vi "Main Tclk.vi"() -> ()   [LabVIEW 2018] (continued)
                                }
                                }
                              }
                            }
                          }
                          n5924 = local write "Status message"("Finishing FIB reheat ..." ("Status message")) -> ()
                          n5925 = local read "Stop Reheat"() -> (w964:bool)
                          n5926 = local read "Stop"() -> (w971:bool)
                          n5927 = Compound Arithmetic op=OR(w967, w971, w964) -> (w969:bool)
                        }
                      }
                      frame #5 {
                        n5928 = local read "Stop Reheat"() -> (w1024:bool)
                        n5929 = case shown="False" w1024 {
                          frame False {
                            n5930 = local read "Api"() -> (w1026:refnum<k7>)
                            n5931 = call "SmartSEM Remote API FIB HV offset removal.vi"("Max offset threshold (V)"=sgl 80.0, "Api"=w1026) -> ("FIB HV matched"=w1025:bool)  [unwired: 8 in, 1 out]
                            n5932 = local write "FIB HV target matched"(w1025) -> ()
                          }
                          frame True {
                          }
                        }
                      }
                      frame #6 {
                        n5933 = local read "Stop Reheat"() -> (w1028:bool)
                        n5934 = case shown="False" w1028 {
                          tunnel: w1029 -> [w1031 w1036]
                          frame False {
                            n5935 = local read "Reheat Output"() -> (w1034:T21)
                            n5936 = local read "FIB Reheat Log Files"() -> (w1033:path)
                            n5937 = local read "Reheat time"() -> (w1032:timestamp)
                            n5938 = local read "Capella HV Data Output"() -> (w1030:T17)
                            n5939 = local write "Status message"("FIB reheat completed" ("Status message")) -> ()
                            n5940 = call "Write FIB reheat log.vi"("Capella HV Data Output"=w1030, "Reheat Output"=w1034, "Reheat time"=w1032, "Machine Type"=w1031, "Log file path"=w1033) -> ()  [unwired: 7 in]
                          }
                          frame True {
                            n5941 = local read "Reheat Output"() -> (w1039:T21)
                            n5942 = local read "FIB Reheat Log Files"() -> (w1038:path)
                            n5943 = local read "Reheat time"() -> (w1037:timestamp)
                            n5944 = local write "Status message"("FIB reheat stopped" ("Status message")) -> ()
                            n5945 = call "Write FIB reheat log.vi"("Reheat Output"=w1039, "Reheat time"=w1037, "Machine Type"=w1036, "Log file path"=w1038) -> ()  [unwired: 8 in]
                          }
                        }
                      }
                    }
                  }
                }
              }
              frame #2 {
                w1041 = u8 0 ("FIB emission below limit counts")
                w1044 = FALSE ("Start Reheat")
                n5946 = local write "Start Reheat"(w1044) -> ()
                n5947 = local write "Stop Reheat"(w1044) -> ()
                n5948 = local write "Turn FIB Gun on"(w1044) -> ()
                n5949 = property on="Request to stop reheat" class="Bool (strict)"("DisabledEnum"=T44."Disabled and Grayed Out" ("Disabled")) -> ()  [unwired: 2 in, 2 out]
                n5950 = local write "FIB emission limit warning armed"(TRUE ("FIB emission limit warning armed")) -> ()
                n5951 = local write "FIB emission below limit counts"(w1041) -> ()
                n5952 = local write "FIB suppressor below limit counts"(w1041) -> ()
                "Reheat completed" <- TRUE ("Reheat completed")
              }
            }
          }
        }
        n5953 = local read "Stop"() -> (w768:bool)
      }
      n5954 = while {
        stop <- w5378 stop-if-true
        n5955 = stacked-sequence {
          tunnel: [_ w5424] -> w5378
          frame #0 {
            n5956 = local read "Spot"() -> (w5381:bool)
            n5957 = shared-variable "My Computer\\Zeiss Library.lvlib\\Spot"(w5381) -> ()  [unwired: 1 in, 1 out]
            n5958 = local read "Machine Type"() -> (w5380:u8)
            n5959 = case shown="True" w5381 {
              tunnel: w5380 -> [_ w5383]
              frame False {
                n5960 = shared-variable ".\\Zeiss Library.lvlib\\FIB spot mode"(FALSE ("FIB spot mode")) -> ()  [unwired: 1 in, 1 out]
              }
              frame True {
                n5961 = stacked-sequence {
                  tunnel: w5383 -> [_ _ _ _ w5405 _ _]
                  frame #0 {
                    w5385 = 5.0 ("Cursor.Cursor Position:Cursor X")
                    w5384 = FALSE ("Unfreeze")
                    w5386 = TRUE ("Realtime Imaging stop")
                    n5962 = shared-variable "My Computer\\Zeiss Library.lvlib\\Realtime Imaging stop"(w5386) -> ()  [unwired: 1 in, 1 out]
                    n5963 = shared-variable ".\\Zeiss Library.lvlib\\FIB spot mode"(w5386) -> ()  [unwired: 1 in, 1 out]
                    n5964 = property on="FIB Imaging" class="Bool (strict)"("DisabledEnum"=T44."Disabled and Grayed Out" ("Disabled")) -> ()  [unwired: 2 in, 2 out]
                    n5965 = property on="FIB Image" class="IntGraph (strict)"() -> ("Width"=w5388:u32, "Height"=w5389:u32)  [unwired: 2 in, 2 out]
                    n5966 = expression code="x/2"(w5388) -> ()  [unwired: 1 out]
                    n5967 = expression code="x/2"(w5389) -> ()  [unwired: 1 out]
                    n5968 = local write "FIB Imaging"(w5384) -> ()
                    n5969 = local write "Unfreeze"(w5384) -> ()
                    n5970 = property on="FIB Image" class="IntGraph (strict)"("Cursor.Cursor X"=w5385, "Cursor.Cursor Y"=w5385) -> ()  [unwired: 2 in, 2 out]
                  }
                  frame #1 {
                    w5390 = -0.99 ("Spot X")
                    n5971 = Wait (ms)(milliseconds to wait=u32 500) -> ()  [unwired: 1 out]
                    n5972 = shared-variable ".\\Zeiss Library.lvlib\\Spot X"(w5390) -> ()  [unwired: 1 in, 1 out]
                    n5973 = shared-variable "My Computer\\Zeiss Library.lvlib\\Spot Z"(w5390) -> ()  [unwired: 1 in, 1 out]
                  }
                  frame #2 {
                    n5974 = local read "FIB HW Config"() -> (w5393:T23)
                    n5975 = local read "FIB Options"() -> (w5397:T33)
                    n5976 = local read "FIB Scan Parameters"() -> (w5392:T32)
                    n5977 = Unbundle By Name(w5397) -> ("Flip x"=w5396:bool, "Flip z"=w5395:bool)
                    n5978 = Bundle("Flip x"=w5396, "Flip z"=w5395) -> (w5394:cluster{"Flip x":bool, "Flip z":bool})  [unwired: 1 in]
                    n5979 = call "FIB spot PXIe-6124.vi"("FIB Scan Parameters"=w5392, "Options"=w5394, "HW Config"=w5393) -> ("error out"=w5399:errorcluster)  [unwired: 8 in]
                    n5980 = Unbundle By Name(w5399) -> ("status"=w5398:bool)
                    n5981 = case shown="True" w5398 {
                      frame False {
                      }
                      frame True {
                        n5982 = local write "Spot"(FALSE ("Spot")) -> ()
                      }
                    }
                  }
                  frame #3 {
                    n5983 = disable-structure shown="Disabled" {
                      frame Disabled {
                        w5404 = TRUE ("Unfreeze")
                        n5984 = local write "FIB Imaging"(w5404) -> ()
                        n5985 = local write "Unfreeze"(w5404) -> ()
                      }
                      frame Enabled {
                      }
                    }
                    n5986 = shared-variable ".\\Zeiss Library.lvlib\\FIB spot mode"(FALSE ("Realtime Imaging stop")) -> ()  [unwired: 1 in, 1 out]
                    n5987 = property on="FIB Imaging" class="Bool (strict)"("DisabledEnum"=T44."Enabled" ("Disabled")) -> ()  [unwired: 2 in, 2 out]
                    n5988 = property on="Spot" class="Bool (strict)"("DisabledEnum"=T44."Disabled and Grayed Out" ("Disabled")) -> ()  [unwired: 2 in, 2 out]
                  }
                  frame #4 {
                    n5989 = case shown="2" w5405 {
                      frame 0, Default {
                      }
                      frame 1 {
                        w5407 = TRUE ("Initialization")
                        n5990 = local read "COM port"() -> (w5406:refnum<visa-resource-name>)
                        n5991 = call "FIB mode.vi"("Initialization"=w5407, "FIB mode"=T10."SEM", "COM port in"=w5406) -> ("COM port out"=w5412:refnum<visa-resource-name>)  [unwired: 7 in, 1 out]
                        n5992 = call "Remcon32 command.vi"("SEM command"="edx 0", "COM port in"=w5412) -> ("COM port out"=w5411:refnum<visa-resource-name>)  [unwired: 6 in, 3 out]
                        n5993 = call "Remcon32 command.vi"("Close session"=w5407, "SEM command"="frez", "COM port in"=w5411) -> ()  [unwired: 5 in, 4 out]
                      }
                      frame 2 {
                        n5994 = local read "Api"() -> (w5413:refnum<k7>)
                        n5995 = call "SmartSEM Remote API set float.vi"("vValue"=sgl 2.0, "lpszParam"="DP_FIB_BLANKER_MODE" ("lpszCommand"), "Api"=w5413) -> ("error out"=w5421:errorcluster, "Api out"=w5420:refnum<k7>)  [unwired: 7 in]
                        n5996 = call "SmartSEM Remote API FIB mode.vi"("error in"=w5421, "FIB mode"=T50."SEM", "Api"=w5420) -> ("error out"=w5417:errorcluster, "Api out"=w5416:refnum<k7>)  [unwired: 7 in]
                        n5997 = invoke class="_EMApi" method="Execute"(reference=w5416, error in=w5417, "lpszCommand"="CMD_FREEZE_ALL") -> ()  [unwired: 1 in, 4 out]
                      }
                    }
                  }
                  frame #5 {
                    n5998 = Wait (ms)(milliseconds to wait=u32 4000) -> ()  [unwired: 1 out]
                  }
                  frame #6 {
                    n5999 = property on="Spot" class="Bool (strict)"("DisabledEnum"=T44."Enabled" ("Disabled")) -> ()  [unwired: 2 in, 2 out]
                  }
                }
              }
            }
          }
          frame #1 {
            n6000 = local read "Stop"() -> (w5424:bool)
          }
        }
        n6001 = Wait Until Next ms Multiple(millisecond multiple=u32 100) -> ()  [unwired: 1 out]
      }
      n6002 = while {
        stop <- w2345 stop-if-true
        n6003 = case shown="True" "Scan xn" {
          tunnel: [w2347 w2348] -> w2345
          frame False {
            n6004 = local read "Stop"() -> (w2347:bool)
          }
          frame True {
            n6005 = while {
              tunnel: [w2351] -> w2348
              stop <- w2353 stop-if-true
              n6006 = stacked-sequence {
                seq-local: [w2355 _ _ _] -> [_ w2371 _ _]
                seq-local: [_ w2370 _ _] -> [_ _ w2377 _]
                seq-local: [_ w2369 _ _] -> [_ _ w2378 _]
                frame #0 {
                  n6007 = local read "Tiled scan inputs"() -> (w2356:T6)
                  n6008 = local read "SEM HW Config"() -> (w2357:T9)
                  n6009 = local read "Detector Information"() -> (w2358:T8)
                  n6010 = local read "SEM Scan Parameters"() -> (w2359:T26)
                  n6011 = local read "SEM Options"() -> (w2360:T27)
                  n6012 = local read "Focus Index Options"() -> (w2354:T28)
                  n6013 = local read "File Information"() -> (w2361:T31)
                  n6014 = local read "Milling para"() -> (w2362:T35)
                  n6015 = Bundle By Name(cluster=w2356, "HW Config"=w2357, "Det Info"=w2358, "SEM Scan Parameters"=w2359, "SEM Options"=w2360, "Focus Index Options"=w2354, "File Information"=w2361, "Milling para"=w2362) -> (w2355:T6)
                }
                frame #1 {
                  n6016 = call "2D scan tiled.vi"("Tiled scan inputs"=w2371) -> ("Image Focus Index Tiled"=w2369:T52, "Image Focus Index Array Tiled"=w2370:T53, "Single scan outputs"=w2374:T54, "8-bit over scale"=w2363:bool[])  [unwired: 5 in, 2 out]
                  n6017 = Unbundle By Name(w2374) -> ("SEM Parameters"=w2373:T13, "Image Focus Index"=w2372:T14)
                  n6018 = Index Array(array=w2363, index #1=0 ("index"), index #2=1 ("index")) -> (element #1=w2366:bool, element #2=w2367:bool)
                  n6019 = local write "SEM Parameters"(w2373) -> ()
                  n6020 = local write "Image Focus Index"(w2372) -> ()
                  n6021 = local write "Det A over scale"(w2366) -> ()
                  n6022 = local write "Det B over scale"(w2367) -> ()
                  n6023 = local write "Status message"("SEM scanning" ("Status message")) -> ()
                }
                frame #2 {
                  n6024 = local read "FI Detector"() -> (w2379:u16)
                  n6025 = case shown="0, Default" w2379 {
                    tunnel: w2378 -> [w2383 w2387 w2391 w2395]
                    tunnel: [w2382 w2384 w2390 w2394] -> w2376
                    tunnel: w2377 -> [w2380 w2386 w2389 w2393]
                    tunnel: [w2381 w2385 w2388 w2392] -> w2375
                    frame 0, Default {
                      n6026 = Unbundle By Name(w2383) -> ("A Img Focus Index"=w2382:sgl[][])
                      n6027 = Unbundle By Name(w2380) -> ("A Img Focus Index array"=w2381:sgl[][][][])
                    }
                    frame 1 {
                      n6028 = Unbundle By Name(w2387) -> ("B Img Focus Index"=w2384:sgl[][])
                      n6029 = Unbundle By Name(w2386) -> ("B Img Focus Index array"=w2385:sgl[][][][])
                    }
                    frame 2 {
                      n6030 = Unbundle By Name(w2391) -> ("C Img Focus Index"=w2390:sgl[][])
                      n6031 = Unbundle By Name(w2389) -> ("C Img Focus Index array"=w2388:sgl[][][][])
                    }
                    frame 3 {
                      n6032 = Unbundle By Name(w2395) -> ("D Img Focus Index"=w2394:sgl[][])
                      n6033 = Unbundle By Name(w2393) -> ("D Img Focus Index array"=w2392:sgl[][][][])
                    }
                  }
                  n6034 = local write "Focus Index array tiled"(w2375) -> ()
                  n6035 = local write "Focus Index tiled"(w2376) -> ()
                }
                frame #3 {
                  n6036 = local read "Scan xn"() -> (w2396:bool)
                  n6037 = case shown="False" w2396 {
                    tunnel: ["SEM scanning pause" ("Status message") "SEM scanning finished" ("Status message")] -> w2397
                    frame True {
                    }
                    frame False {
                    }
                  }
                  n6038 = local write "Status message"(w2397) -> ()
                  n6039 = Wait (ms)(milliseconds to wait=u32 1000) -> ()  [unwired: 1 out]
                }
              }
              n6040 = Wait Until Next ms Multiple(millisecond multiple=u32 100) -> ()  [unwired: 1 out]
              n6041 = local read "Scan xn"() -> (w2352:bool)
              n6042 = Not(x=w2352) -> (.not. x?=w2350:bool)
              n6043 = local read "Stop"() -> (w2351:bool)
              n6044 = Or(x=w2350, y=w2351) -> (x .or. y?=w2353:bool)
            }
          }
        }
        n6045 = Wait Until Next ms Multiple(millisecond multiple=u32 100) -> ()  [unwired: 1 out]
      }
      n6046 = while {
        stop <- w2927 stop-if-true
        w2934 = -1.0 ("lower limit")
        w2935 = 1.0 ("upper limit")
        n6047 = property on="FIB Image" class="IntGraph (strict)"() -> ("Cursor.Cursor X"=w2929:dbl, "Width"=w2928:u32, "Cursor.Cursor Y"=w2931:dbl, "Height"=w2930:u32)  [unwired: 2 in, 2 out]
        n6048 = local read "Stop"() -> (w2927:bool)
        n6049 = Wait Until Next ms Multiple(millisecond multiple=u32 10) -> ()  [unwired: 1 out]
        n6050 = Not(x=w2927) -> (.not. x?=w2925:bool)
        n6051 = expression code="x/2"(w2928) -> (w2933:u32)
        n6052 = expression code="x/2"(w2930) -> (w2932:u32)
        n6053 = Compound Arithmetic op=AND("Spot", w2925) -> (w2945:bool)
        n6054 = shared-variable "My Computer\\Zeiss Library.lvlib\\Milling Manual Pause"("Mill Manual Pause") -> (error out=w2924:errorcluster)  [unwired: 1 in]
        n6055 = shared-variable "My Computer\\Zeiss Library.lvlib\\Milling Stop"("Mill Stop", error in=w2924) -> (error out=w2923:errorcluster)
        n6056 = shared-variable ".\\Zeiss Library.lvlib\\FIB beam blank"("Beam blanked", error in=w2923) -> (error out=w2922:errorcluster)
        n6057 = property on="FIB Image" class="IntGraph (strict)"("Cursor.Visible"="Spot") -> ()  [unwired: 2 in, 2 out]
        n6058 = Subtract(x=w2929, y=w2933) -> (x-y=w2941:dbl)
        n6059 = Subtract(x=w2931, y=w2932) -> (x-y=w2940:dbl)
        n6060 = Divide(x=w2941, y=w2933) -> (x/y=w2939:dbl)
        n6061 = Divide(x=w2940, y=w2932) -> (x/y=w2936:dbl)
        n6062 = In Range and Coerce(upper limit=w2935, x=w2939, lower limit=w2934) -> (coerced(x)=w2938:dbl)  [unwired: 1 out]
        n6063 = In Range and Coerce(upper limit=w2935, x=w2936, lower limit=w2934) -> (coerced(x)=w2937:dbl)  [unwired: 1 out]
        n6064 = shared-variable ".\\Zeiss Library.lvlib\\Spot X"(w2938, error in=w2922) -> (error out=w2921:errorcluster)
        n6065 = shared-variable "My Computer\\Zeiss Library.lvlib\\Spot Z"(w2937, error in=w2921) -> (error out=w2920:errorcluster)
        n6066 = shared-variable ".\\Zeiss Library.lvlib\\FIB spot mode"(w2945, error in=w2920) -> ()  [unwired: 1 out]
      }
      n6067 = while {
        stop <- w5362 stop-if-true
        n6068 = case shown="True" "Mill" {
          frame False {
            n6069 = property on="FIB Imaging" class="Bool (strict)"("DisabledEnum"=T44."Enabled" ("Disabled")) -> ()  [unwired: 2 in, 2 out]
          }
          frame True {
            n6070 = stacked-sequence {
              frame #0 {
                w5365 = FALSE ("Freeze")
                n6071 = local write "Unfreeze"(w5365) -> ()
                n6072 = local write "Mill Manual Pause"(w5365) -> ()
                n6073 = local write "Mill Stop"(w5365) -> ()
              }
              frame #1 {
                n6074 = Wait (ms)(milliseconds to wait=u32 500) -> ()  [unwired: 1 out]
              }
              frame #2 {
                n6075 = local read "FIB HW Config"() -> (w5371:T23)
                n6076 = local read "FIB Scan Parameters"() -> (w5370:T32)
                n6077 = local read "FIB Options"() -> (w5375:T33)
                n6078 = local read "Machine Type"() -> (w5368:u8)
                n6079 = Unbundle By Name(w5375) -> ("Flip x"=w5374:bool, "Flip z"=w5373:bool)
                n6080 = local read "COM port"() -> (w5369:refnum<visa-resource-name>)
                n6081 = Bundle("Flip x"=w5374, "Flip z"=w5373) -> (w5372:cluster{"Flip x":bool, "Flip z":bool})  [unwired: 1 in]
                n6082 = call "FIB trapezoidal mill PXIe-6124.vi"("Machine Type"=w5368, "COM port"=w5369, "Milling para"="Milling para", "Options"=w5372, "FIB Scan Parameters"=w5370, "HW Config"=w5371) -> ()  [unwired: 2 in, 4 out]
              }
              frame #3 {
                n6083 = shared-variable "My Computer\\Zeiss Library.lvlib\\Milling Line Paused"(TRUE ("Rect Milling Line Paused")) -> ()  [unwired: 1 in, 1 out]
                n6084 = local write "Mill"(FALSE ("Mill")) -> ()
              }
            }
          }
        }
        n6085 = Wait Until Next ms Multiple(millisecond multiple=u32 100) -> ()  [unwired: 1 out]
        n6086 = local read "Stop"() -> (w5362:bool)
      }
      n6087 = while {
        stop <- w1769 stop-if-true
        n6088 = Wait Until Next ms Multiple(millisecond multiple=u32 100) -> ()  [unwired: 1 out]
        n6089 = case shown="True" "Enable logging" {
          frame False {
          }
          frame True {
            n6090 = stacked-sequence {
              frame #0 {
                n6091 = Get Date/Time In Seconds() -> (seconds since 1Jan1904=w1775:timestamp)
                n6092 = Reciprocal(x="Sample rate (Hz)") -> (1/x=w1772:dbl)
                n6093 = To Double Precision Float(number=w1775) -> (double precision float=w1774:dbl)
                n6094 = property on="Measurements" class="WFChart (strict)"("History Data"=dbl[][] [], "XScale.Offset"=w1774, "XScale.Multiplier"=w1772) -> ()  [unwired: 2 in, 2 out]
              }
              frame #1 {
                w1790 = 10123 items=["Finite Samples"=10178, "Continuous Samples"=10123, "Hardware Timed Single Point"=12522] ("sample mode")
                n6095 = local read "Sample rate (Hz)"() -> (w1780:dbl)
                n6096 = local read "Active logging channels"() -> (w1779:string)
                n6097 = call-poly <vilib>:"DAQmx Create Virtual Channel.vi"("physical channels"=w1779) -> ("task out"=w1789:refnum<k21>, "error out"=w1788:errorcluster)  [unwired: 13 in]
                n6098 = call-poly <vilib>:"DAQmx Timing.vi"("task/channels in"=w1789, "sample mode"=w1790, "rate"=w1780, "error in"=w1788) -> ("task out"=w1777:refnum<k21>, "error out"=w1786:errorcluster)  [unwired: 10 in]
                n6099 = local read "Machine Type"() -> (w1776:u8)
                n6100 = call <vilib>:"DAQmx Configure Input Buffer.vi"("task/channels in"=w1777, "buffer size (in samples per channel)"=u32 1000000, "error in"=w1786) -> ("task out"=w1787:refnum<k21>, "error out"=w1785:errorcluster)  [unwired: 11 in]
                n6101 = call <vilib>:"DAQmx Start Task.vi"("task/channels in"=w1787, "error in"=w1785) -> ("task out"=w1782:refnum<k21>, "error out"=w1781:errorcluster)  [unwired: 12 in]
                n6102 = while {
                  tunnel: w1781 -> [w1820]
                  tunnel: w1782 -> [w1819]
                  tunnel: [w1818] -> w1783
                  tunnel: [w1817] -> w1784
                  tunnel: w1776 -> [w1795]
                  stop <- w1813 stop-if-true
                  n6103 = local read "Faraday Cup before mill"() -> (w1802:sgl)
                  n6104 = call-poly <vilib>:"DAQmx Read.vi"("task/channels in"=w1819, "number of samples per channel"="Samples size", "error in"=w1820) -> ("task out"=w1818:refnum<k21>, "data"=w1811:dbl[][], "error out"=w1817:errorcluster)  [unwired: 10 in]
                  n6105 = To Single Precision Float(number=w1811) -> (single precision float=w1810:sgl[][])
                  n6106 = expression code="x*10"(w1810) -> (w1793:sgl[][])
                  n6107 = case shown="2" w1795 {
                    tunnel: w1793 -> [w1821 w1824]
                    tunnel: "Samples size" -> [_ w1823]
                    tunnel: [w1821 w1822] -> w1792
                    frame 0, Default {
                    }
                    frame 2 {
                      n6108 = local read "Api"() -> (w1825:refnum<k7>)
                      n6109 = call "SmartSEM Remote API FIB Faraday cup.vi"("Api"=w1825) -> ("FIB Faraday Cup (nA)"=w1826:sgl)  [unwired: 8 in, 2 out]
                      n6110 = Initialize Array(w1826, w1823) -> (w1827:sgl[])
                      n6111 = Replace Array Subset(array=w1824, new element=w1827) -> (w1822:sgl[][])  [unwired: 2 in]
                    }
                  }
                  "Measurements" <- w1792
                  n6112 = call "2D Array Decimate.vi"("x decimating factor"="Samples size", "Input 2D Array"=w1792) -> ("output array"=w1809:dbl[][])  [unwired: 7 in, 2 out]
                  n6113 = To Single Precision Float(number=w1809) -> (single precision float=w1808:sgl[][])
                  n6114 = Index Array(array=w1808, index (col)=0 ("disabled index (col)")) -> (element=w1804:sgl[])  [unwired: 1 in]
                  n6115 = Index Array(array=w1804, index #1=3 ("index"), index #2=2 ("index"), index #3=1 ("index"), index #4=0 ("index")) -> (element #1=→"BD2 RT":sgl, element #2=w1801:sgl, element #3=→"Specimen RT":sgl, element #4=→"Faraday Cup RT":sgl)
                  "BD1 RT" <- w1801
                  n6116 = local read "Enable logging"() -> (w1816:bool)
                  n6117 = Subtract(x=w1802, y=w1801) -> (x-y=w1805:sgl)
                  n6118 = local read "Stop"() -> (w1814:bool)
                  n6119 = Build Array (concatenate)(w1804, w1805) -> (w1803:sgl[])
                  n6120 = shared-variable ".\\Zeiss Library.lvlib\\Logs"(w1803) -> ()  [unwired: 1 in, 1 out]
                  n6121 = Not(x=w1816) -> (.not. x?=w1815:bool)
                  n6122 = Or(x=w1815, y=w1814) -> (x .or. y?=w1813:bool)
                }
                n6123 = call <vilib>:"DAQmx Clear Task.vi"("task in"=w1783, "error in"=w1784) -> ("error out"=w1778:errorcluster)  [unwired: 13 in]
                n6124 = call <vilib>:"General Error Handler.vi"("error in (no error)"=w1778) -> ()  [unwired: 10 in, 5 out]
              }
            }
          }
        }
        n6125 = local read "Stop"() -> (w1769:bool)
      }
      n6126 = while {
        shift-right: [w1829] -> _
        shift-left: _ -> [w1828]
        stop <- w1831 stop-if-true
        n6127 = stacked-sequence {
          tunnel: [_ _ _ _ _ _ _ _ _ _ _ _ _ _ _ _ w2138 _ _ _ _ _ _ _ _ _] -> w1829
          tunnel: w1828 -> [_ _ _ _ _ _ _ _ _ _ _ _ _ _ _ _ w2139 w2156 w2174 _ _ _ _ _ _ _]
          frame #0 {
            n6128 = local read "FIB slice #"() -> (w1836:u32)
            n6129 = Not Equal To 0?(x="Images per Auto Optimization") -> (x != 0?=w1833:bool)
            n6130 = Not Equal To 0?(x=w1836) -> (x != 0?=w1837:bool)
            n6131 = Compound Arithmetic op=AND("Auto Optimzation", w1833, w1837) -> (w1832:bool)
            n6132 = case shown="True" w1832 {
              frame False {
              }
              frame True {
                n6133 = local read "WD array tiled"() -> (w1843:sgl[][][])
                n6134 = local read "StigX array tiled"() -> (w1841:sgl[][][])
                n6135 = local read "StigY array tiled"() -> (w1840:sgl[][][])
                n6136 = local read "AF Steps"() -> (w1859:u8)
                n6137 = local read "FIB slice #"() -> (w1853:u32)
                n6138 = local read "Images per Auto Optimization"() -> (w1857:u16)
                n6139 = Empty Array?(array=w1843) -> (empty?=w1842:bool)
                n6140 = Empty Array?(array=w1841) -> (empty?=w1839:bool)
                n6141 = Empty Array?(array=w1840) -> (empty?=w1838:bool)
                n6142 = local read "AF Success tiled"() -> (w1845:bool[][])
                n6143 = Increment(x=w1859) -> (x+1=w1858:u8)
                n6144 = And(x=w1839, y=w1838) -> (x .and. y?=w1846:bool)
                n6145 = local read "Auto Stig"() -> (w1850:bool)
                n6146 = local read "Auto Align"() -> (w1848:bool)
                n6147 = Quotient & Remainder(x=w1853, y=w1857) -> (x-y*floor(x/y)=w1860:u32)  [unwired: 1 out]
                n6148 = And Array Elements(Boolean array=w1845) -> (logical AND=w1844:bool)
                n6149 = Equal?(x=w1858, y=w1860) -> (x = y?=w1852:bool)
                n6150 = Not Equal To 0?(x=w1853) -> (x != 0?=w1854:bool)
                n6151 = Equal To 0?(x=w1860) -> (x = 0?=w1855:bool)
                n6152 = Not(x=w1850) -> (.not. x?=w1849:bool)
                n6153 = Not(x=w1848) -> (.not. x?=w1847:bool)
                n6154 = Compound Arithmetic op=AND(w1842, w1844, w1852, w1847) -> (w1851:bool)
                n6155 = Compound Arithmetic op=AND(w1854, w1855, w1846, w1849, w1847) -> (w1856:bool)
                n6156 = case shown="True" w1851 {
                  frame False {
                  }
                  frame True {
                    n6157 = local write "Auto Stig"(TRUE ("Auto Focus")) -> ()
                  }
                }
                n6158 = case shown="True" w1856 {
                  frame False {
                  }
                  frame True {
                    n6159 = local write "Auto Focus"(TRUE ("Auto Focus")) -> ()
                  }
                }
              }
            }
          }
          frame #1 {
            n6160 = local read "Email Alert Recipients"() -> (w1866:string[])
            n6161 = local read "Mail server"() -> (w1867:string)
            n6162 = local read "Hardware Configuration"() -> (w1869:T25)
            n6163 = local read "Email Log Files"() -> (w1863:path)
            n6164 = Unbundle By Name(w1869) -> ("Machine ID"=w1868:string)
            n6165 = call "Email alert.vi"("Email log file path"=w1863, "Send email"="E-mail test", "Machine ID"=w1868, "Mail server"=w1867, "Alarm message"="E-mail test", "Recipents"=w1866) -> ()  [unwired: 6 in]
            n6166 = case shown="True" "E-mail test" {
              frame False {
              }
              frame True {
                n6167 = stacked-sequence {
                  frame #0 {
                    n6168 = Wait (ms)(milliseconds to wait=u32 200) -> ()  [unwired: 1 out]
                  }
                  frame #1 {
                    n6169 = local write "E-mail test"(FALSE ("E-mail test")) -> ()
                  }
                }
              }
            }
          }
          frame #2 {
            n6170 = local read "Machine Type"() -> (w1880:u8)
            n6171 = case shown="2" w1880 {
              tunnel: [w1890 w1892 w1894] -> w1881
              frame 0, Default {
                n6172 = local read "HV Data Output"() -> (w1891:T18)
                n6173 = Unbundle By Name(w1891) -> ("Emission (uA)"=w1890:sgl)
              }
              frame 1 {
                n6174 = local read "FIB Parameters"() -> (w1893:T19)
                n6175 = Unbundle By Name(w1893) -> ("FIB emission (uA)"=w1892:sgl)
              }
              frame 2 {
                n6176 = local read "Capella HV Data Output"() -> (w1895:T17)
                n6177 = Unbundle By Name(w1895) -> ("Emission Actual (uA)"=w1894:sgl)
              }
            }
            n6178 = local read "Alert Settings"() -> (w1878:T36)
            n6179 = local read "FIB"() -> (w1872:bool)
            n6180 = local read "FIB emission limit warning active"() -> (w1883:bool)
            n6181 = local read "FIB emission limit warning armed"() -> (w1884:bool)
            n6182 = Unbundle By Name(w1878) -> ("FIB emission warning"=w1877:bool)
            n6183 = Format Into String(format string="%4.2f", w1881) -> (resulting string=w1882:string)  [unwired: 2 in, 1 out]
            n6184 = Concatenate Strings("FIB emission reached ", w1882, "uA" ("resulting string")) -> (w1879:string)
            n6185 = case shown="True" w1883 {
              frame False {
              }
              frame True {
                n6186 = stacked-sequence {
                  frame #0 {
                    n6187 = Wait (ms)(milliseconds to wait=u32 500) -> ()  [unwired: 1 out]
                  }
                  frame #1 {
                    "FIB emission limit warning armed" <- FALSE ("3D image paused active bypass")
                  }
                }
              }
            }
            n6188 = local read "Email Alert Recipients"() -> (w1885:string[])
            n6189 = local read "Mail server"() -> (w1886:string)
            n6190 = local read "Hardware Configuration"() -> (w1889:T25)
            n6191 = local read "Email Log Files"() -> (w1876:path)
            n6192 = Compound Arithmetic op=AND(w1872, w1883, w1884, w1877) -> (w1888:bool)
            n6193 = Unbundle By Name(w1889) -> ("Machine ID"=w1887:string)
            n6194 = call "Email alert.vi"("Email log file path"=w1876, "Send email"=w1888, "Machine ID"=w1887, "Mail server"=w1886, "Alarm message"=w1879, "Recipents"=w1885) -> ()  [unwired: 6 in]
          }
          frame #3 {
            n6195 = local read "Alert Settings"() -> (w1902:T36)
            n6196 = local read "FIB"() -> (w1898:bool)
            n6197 = Unbundle By Name(w1902) -> ("FIB CL current alarm"=w1901:bool)
            n6198 = local read "FIB CL I alarm active"() -> (w1903:bool)
            n6199 = local read "Email Alert Recipients"() -> (w1905:string[])
            n6200 = local read "Mail server"() -> (w1906:string)
            n6201 = local read "Hardware Configuration"() -> (w1908:T25)
            n6202 = local read "Email Log Files"() -> (w1899:path)
            n6203 = Unbundle By Name(w1908) -> ("Machine ID"=w1907:string)
            n6204 = Compound Arithmetic op=AND(w1898, w1901, w1903) -> (w1900:bool)
            n6205 = call "Email alert.vi"("Email log file path"=w1899, "Send email"=w1900, "Machine ID"=w1907, "Mail server"=w1906, "Alarm message"="FIB CL current out of bound", "Recipents"=w1905) -> ()  [unwired: 6 in]
            n6206 = case shown="True" w1900 {
              frame False {
              }
              frame True {
                n6207 = stacked-sequence {
                  frame #0 {
                    n6208 = Wait (ms)(milliseconds to wait=u32 200) -> ()  [unwired: 1 out]
                  }
                  frame #1 {
                    n6209 = local write "FIB CL I alarm active"(FALSE ("E-mail test")) -> ()
                    n6210 = local write "FIB CL I out of bound counts"(u8 0 ("Specimen I out of bound counts")) -> ()
                  }
                }
              }
            }
          }
          frame #4 {
            n6211 = local read "Alert Settings"() -> (w1916:T36)
            n6212 = local read "FIB"() -> (w1912:bool)
            n6213 = Unbundle By Name(w1916) -> ("Beam Dump 1 alarm"=w1915:bool)
            n6214 = local read "Beam dump at zero"() -> (w1917:bool)
            n6215 = local read "Email Alert Recipients"() -> (w1919:string[])
            n6216 = local read "Mail server"() -> (w1920:string)
            n6217 = local read "Hardware Configuration"() -> (w1922:T25)
            n6218 = local read "Email Log Files"() -> (w1913:path)
            n6219 = Compound Arithmetic op=AND(w1912, w1915, w1917) -> (w1914:bool)
            n6220 = Unbundle By Name(w1922) -> ("Machine ID"=w1921:string)
            n6221 = call "Email alert.vi"("Email log file path"=w1913, "Send email"=w1914, "Machine ID"=w1921, "Mail server"=w1920, "Alarm message"="Beam dump current at or near zero", "Recipents"=w1919) -> ()  [unwired: 6 in]
            n6222 = case shown="True" w1914 {
              frame False {
              }
              frame True {
                n6223 = stacked-sequence {
                  frame #0 {
                    n6224 = Wait (ms)(milliseconds to wait=u32 200) -> ()  [unwired: 1 out]
                  }
                  frame #1 {
                    n6225 = local write "Beam dump at zero"(FALSE ("E-mail test")) -> ()
                  }
                }
              }
            }
          }
          frame #5 {
            n6226 = local read "Faraday Cup < Milling current"() -> (w1926:bool)
            n6227 = local read "FIB"() -> (w1925:bool)
            n6228 = local read "Email Alert Recipients"() -> (w1930:string[])
            n6229 = local read "Mail server"() -> (w1931:string)
            n6230 = local read "Hardware Configuration"() -> (w1933:T25)
            n6231 = local read "Email Log Files"() -> (w1928:path)
            n6232 = Unbundle By Name(w1933) -> ("Machine ID"=w1932:string)
            n6233 = Compound Arithmetic op=AND(w1925, w1926) -> (w1927:bool)
            n6234 = call "Email alert.vi"("Email log file path"=w1928, "Send email"=w1927, "Machine ID"=w1932, "Mail server"=w1931, "Alarm message"="Faraday cup current < Milling current", "Recipents"=w1930) -> ()  [unwired: 6 in]
            n6235 = case shown="True" w1927 {
              frame False {
              }
              frame True {
                n6236 = stacked-sequence {
                  frame #0 {
                    n6237 = Wait (ms)(milliseconds to wait=u32 200) -> ()  [unwired: 1 out]
                  }
                  frame #1 {
                    n6238 = local write "Faraday Cup < Milling current"(FALSE ("E-mail test")) -> ()
                  }
                }
              }
            }
          }
          frame #6 {
            n6239 = local read "SEM Status"() -> (w1942:T12)
            n6240 = Unbundle By Name(w1942) -> ("SEM Spec. I (nA)"=w1939:sgl)
            n6241 = local read "FIB"() -> (w1938:bool)
            n6242 = local read "SEM Spec. I spike"() -> (w1937:bool)
            n6243 = local read "Email Alert Recipients"() -> (w1947:string[])
            n6244 = local read "Mail server"() -> (w1948:string)
            n6245 = local read "Hardware Configuration"() -> (w1950:T25)
            n6246 = local read "Email Log Files"() -> (w1946:path)
            n6247 = Format Into String(format string="%#g", w1939) -> (resulting string=w1940:string)  [unwired: 2 in, 1 out]
            n6248 = Compound Arithmetic op=AND(w1938, w1937) -> (w1936:bool)
            n6249 = Unbundle By Name(w1950) -> ("Machine ID"=w1949:string)
            n6250 = Concatenate Strings("SEM specimen current spiked to " ("Alarm message"), w1940, " nA" ("Alarm message")) -> (w1944:string)
            n6251 = call "Email alert.vi"("Email log file path"=w1946, "Send email"=w1936, "Machine ID"=w1949, "Mail server"=w1948, "Alarm message"=w1944, "Recipents"=w1947) -> ()  [unwired: 6 in]
            n6252 = case shown="True" w1936 {
              frame False {
              }
              frame True {
                n6253 = stacked-sequence {
                  frame #0 {
                    n6254 = Wait (ms)(milliseconds to wait=u32 200) -> ()  [unwired: 1 out]
                  }
                  frame #1 {
                    n6255 = local write "SEM Spec. I spike"(FALSE ("E-mail test")) -> ()
                  }
                }
              }
            }
          }
          frame #7 {
            n6256 = local read "Milling Z voltage (V)"() -> (w1956:sgl)
            n6257 = local read "FIB"() -> (w1955:bool)
            n6258 = local read "Milling Z voltage spike"() -> (w1954:bool)
            n6259 = local read "Email Alert Recipients"() -> (w1963:string[])
            n6260 = local read "Mail server"() -> (w1964:string)
            n6261 = local read "Hardware Configuration"() -> (w1966:T25)
            n6262 = local read "Email Log Files"() -> (w1962:path)
            n6263 = Format Into String(format string="%#g", w1956) -> (resulting string=w1957:string)  [unwired: 2 in, 1 out]
            n6264 = Unbundle By Name(w1966) -> ("Machine ID"=w1965:string)
            n6265 = Compound Arithmetic op=AND(w1955, w1954) -> (w1953:bool)
            n6266 = Concatenate Strings("Milling Z voltage spiked to " ("Alarm message"), w1957, " V" ("Alarm message")) -> (w1960:string)
            n6267 = call "Email alert.vi"("Email log file path"=w1962, "Send email"=w1953, "Machine ID"=w1965, "Mail server"=w1964, "Alarm message"=w1960, "Recipents"=w1963) -> ()  [unwired: 6 in]
            n6268 = case shown="True" w1953 {
              frame False {
              }
              frame True {
                n6269 = stacked-sequence {
                  frame #0 {
                    n6270 = Wait (ms)(milliseconds to wait=u32 200) -> ()  [unwired: 1 out]
                  }
                  frame #1 {
                    n6271 = local write "Milling Z voltage spike"(FALSE ("E-mail test")) -> ()
                  }
                }
              }
            }
          }
          frame #8 {
            n6272 = local read "Alert Settings"() -> (w1973:T36)
            n6273 = local read "FIB"() -> (w1969:bool)
            n6274 = Unbundle By Name(w1973) -> ("EHT off alarm"=w1972:bool)
            n6275 = local read "EHT off"() -> (w1974:bool)
            n6276 = local read "Email Alert Recipients"() -> (w1976:string[])
            n6277 = local read "Mail server"() -> (w1977:string)
            n6278 = local read "Hardware Configuration"() -> (w1979:T25)
            n6279 = local read "Email Log Files"() -> (w1970:path)
            n6280 = Compound Arithmetic op=AND(w1969, w1972, w1974) -> (w1971:bool)
            n6281 = Unbundle By Name(w1979) -> ("Machine ID"=w1978:string)
            n6282 = call "Email alert.vi"("Email log file path"=w1970, "Send email"=w1971, "Machine ID"=w1978, "Mail server"=w1977, "Alarm message"="EHT was off", "Recipents"=w1976) -> ()  [unwired: 6 in]
            n6283 = case shown="True" w1971 {
              frame False {
              }
              frame True {
                n6284 = stacked-sequence {
                  frame #0 {
                    n6285 = Wait (ms)(milliseconds to wait=u32 200) -> ()  [unwired: 1 out]
                  }
                  frame #1 {
                    n6286 = local write "EHT off"(FALSE ("E-mail test")) -> ()
                  }
                }
              }
            }
          }
          frame #9 {
            n6287 = local read "Alert Settings"() -> (w1986:T36)
            n6288 = local read "FIB"() -> (w1982:bool)
            n6289 = local read "Det A over scale"() -> (w1984:bool)
            n6290 = local read "Email Alert Recipients"() -> (w1989:string[])
            n6291 = local read "Mail server"() -> (w1990:string)
            n6292 = local read "Hardware Configuration"() -> (w1992:T25)
            n6293 = local read "Email Log Files"() -> (w1987:path)
            n6294 = Unbundle By Name(w1986) -> ("Detector over scale warning"=w1985:bool)
            n6295 = Unbundle By Name(w1992) -> ("Machine ID"=w1991:string)
            n6296 = Compound Arithmetic op=AND(w1982, w1985, w1984) -> (w1983:bool)
            n6297 = call "Email alert.vi"("Email log file path"=w1987, "Send email"=w1983, "Machine ID"=w1991, "Mail server"=w1990, "Alarm message"="Detector A over scale", "Recipents"=w1989) -> ()  [unwired: 6 in]
            n6298 = case shown="True" w1983 {
              frame False {
              }
              frame True {
                n6299 = stacked-sequence {
                  frame #0 {
                    n6300 = Wait (ms)(milliseconds to wait=u32 200) -> ()  [unwired: 1 out]
                  }
                  frame #1 {
                    n6301 = local write "Det A over scale"(FALSE ("E-mail test")) -> ()
                  }
                }
              }
            }
          }
          frame #10 {
            n6302 = local read "Alert Settings"() -> (w1999:T36)
            n6303 = local read "FIB"() -> (w1995:bool)
            n6304 = local read "Email Alert Recipients"() -> (w2002:string[])
            n6305 = local read "Mail server"() -> (w2003:string)
            n6306 = local read "Hardware Configuration"() -> (w2005:T25)
            n6307 = local read "Email Log Files"() -> (w2000:path)
            n6308 = local read "Det B over scale"() -> (w1997:bool)
            n6309 = Unbundle By Name(w1999) -> ("Detector over scale warning"=w1998:bool)
            n6310 = Unbundle By Name(w2005) -> ("Machine ID"=w2004:string)
            n6311 = Compound Arithmetic op=AND(w1995, w1998, w1997) -> (w1996:bool)
            n6312 = call "Email alert.vi"("Email log file path"=w2000, "Send email"=w1996, "Machine ID"=w2004, "Mail server"=w2003, "Alarm message"="Detector B over scale", "Recipents"=w2002) -> ()  [unwired: 6 in]
            n6313 = case shown="True" w1996 {
              frame False {
              }
              frame True {
                n6314 = stacked-sequence {
                  frame #0 {
                    n6315 = Wait (ms)(milliseconds to wait=u32 200) -> ()  [unwired: 1 out]
                  }
                  frame #1 {
                    n6316 = local write "Det B over scale"(FALSE ("E-mail test")) -> ()
                  }
                }
              }
            }
          }
          frame #11 {
            n6317 = local read "Alert Settings"() -> (w2010:T36)
            n6318 = local read "3D image paused active"() -> (w2013:bool)
            n6319 = local read "3D image paused armed"() -> (w2011:bool)
            n6320 = local read "Hardware Configuration"() -> (w2018:T25)
            n6321 = local read "Email Log Files"() -> (w2008:path)
            n6322 = Unbundle By Name(w2010) -> ("3D imaging paused alarm"=w2009:bool)
            n6323 = Unbundle By Name(w2018) -> ("Machine ID"=w2014:string)
            n6324 = case shown="True" w2013 {
              frame False {
              }
              frame True {
                n6325 = stacked-sequence {
                  frame #0 {
                    n6326 = Wait (ms)(milliseconds to wait=u32 500) -> ()  [unwired: 1 out]
                  }
                  frame #1 {
                    w2020 = FALSE ("3D image paused active bypass")
                    n6327 = local write "3D image paused active"(w2020) -> ()
                    "3D image paused armed" <- w2020
                  }
                }
              }
            }
            n6328 = Compound Arithmetic op=AND(w2013, w2011, w2009) -> (w2012:bool)
            n6329 = call "Email alert.vi"("Email log file path"=w2008, "Send email"=w2012, "Machine ID"=w2014, "Mail server"="Mail server", "Alarm message"="3D imaging paused", "Recipents"="Email Alert Recipients") -> ()  [unwired: 6 in]
          }
          frame #12 {
            n6330 = local read "Alert Settings"() -> (w2023:T36)
            n6331 = local read "Email Alert Recipients"() -> (w2028:string[])
            n6332 = local read "SW error warning active"() -> (w2024:bool)
            n6333 = local read "SW error warning armed"() -> (w2025:bool)
            n6334 = local read "Mail server"() -> (w2029:string)
            n6335 = local read "Hardware Configuration"() -> (w2031:T25)
            n6336 = local read "Email Log Files"() -> (w2021:path)
            n6337 = Unbundle By Name(w2023) -> ("SW error warning"=w2022:bool)
            n6338 = Unbundle By Name(w2031) -> ("Machine ID"=w2030:string)
            n6339 = Compound Arithmetic op=AND(w2024, w2025, w2022) -> (w2026:bool)
            n6340 = call "Email alert.vi"("Email log file path"=w2021, "Send email"=w2026, "Machine ID"=w2030, "Mail server"=w2029, "Alarm message"="Software timeout error", "Recipents"=w2028) -> ()  [unwired: 6 in]
            n6341 = case shown="True" w2024 {
              frame False {
              }
              frame True {
                n6342 = stacked-sequence {
                  frame #0 {
                    n6343 = Wait (ms)(milliseconds to wait=u32 500) -> ()  [unwired: 1 out]
                  }
                  frame #1 {
                    w2033 = FALSE ("3D image paused active bypass")
                    n6344 = local write "SW error warning active"(w2033) -> ()
                    "SW error warning armed" <- w2033
                  }
                }
              }
            }
          }
          frame #13 {
            n6345 = local read "Machine Type"() -> (w2034:u8)
            n6346 = case shown="2" w2034 {
              tunnel: [w2050 w2064] -> w2037
              frame 0, Default {
                w2045 = "%#g" ("format string")
                n6347 = local read "Actual Reheat Parameters"() -> (w2058:T1)
                n6348 = local read "HV Data Output"() -> (w2049:T18)
                n6349 = Unbundle By Name(w2049) -> ("Tip Lifetime (hr)"=w2048:sgl)
                n6350 = Unbundle By Name(w2058) -> ("Filament I (A)"=w2057:sgl, "Reheat time (s)"=w2056:sgl)
                n6351 = Format Into String(format string=w2045, w2057) -> (resulting string=w2054:string)  [unwired: 2 in, 1 out]
                n6352 = Format Into String(format string="%d", w2048) -> (resulting string=w2046:string)  [unwired: 2 in, 1 out]
                n6353 = Format Into String(format string=w2045, w2056) -> (resulting string=w2052:string)  [unwired: 2 in, 1 out]
                n6354 = Concatenate Strings("FIB lifetime = " ("Alarm message"), w2046, " hr, FIB reheat started, " ("Alarm message"), w2054, " A for " ("string"), w2052, " s" ("string")) -> (w2050:string)
              }
              frame 2 {
                n6355 = local read "Capella HV Data Output"() -> (w2063:T17)
                n6356 = Unbundle By Name(w2063) -> ("Tip Lifetime (uAhr)"=w2062:sgl)
                n6357 = Format Into String(format string="%d", w2062) -> (resulting string=w2060:string)  [unwired: 2 in, 1 out]
                n6358 = Concatenate Strings("FIB lifetime = " ("Alarm message"), w2060, " uAhr, FIB reheat started" ("Alarm message")) -> (w2064:string)
              }
            }
            n6359 = local read "Mail server"() -> (w2041:string)
            n6360 = local read "Hardware Configuration"() -> (w2043:T25)
            n6361 = local read "Send reheat start email"() -> (w2035:bool)
            n6362 = local read "Reheat warning armed"() -> (w2038:bool)
            n6363 = local read "Email Alert Recipients"() -> (w2040:string[])
            n6364 = Unbundle By Name(w2043) -> ("Machine ID"=w2042:string)
            n6365 = Compound Arithmetic op=AND(w2035, w2038) -> (w2039:bool)
            n6366 = local read "Email Log Files"() -> (w2036:path)
